vi "testD.vi"(11 "Event Registration Refnum":T1) -> ()   [LabVIEW 2015]
uses:
  D refnum.ctl
panel:
  out "Boolean":bool
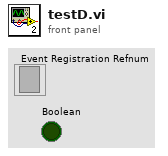
[diagram p1: front panel]
types:
  T1 = typedef "D refnum.ctl" = refnum<event-registration>
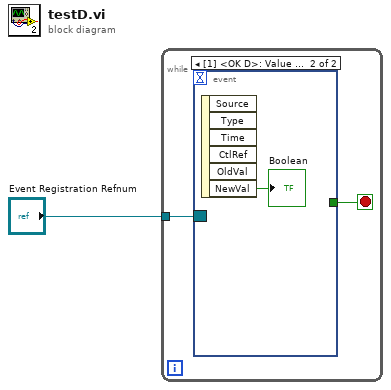
[diagram p0: block diagram]
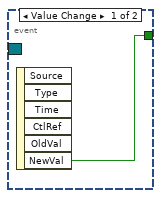
[diagram p2: hidden frame]
diagram:
  n1 = while {
    tunnel: "Event Registration Refnum" -> [w2]
    stop <- w3 stop-if-true
    n2 = event shown="[1] <OK D>: Value Change" {
      selector: w2 -> [_ _]
      dyn-events: _ -> [_ _]
      timeout: _ -> [_ _]
      tunnel: [w4 _] -> w3
      event Value Change {
        n3 = event-data() -> ("NewVal"=w4:bool)  [unwired: 1 in, 5 out]
      }
      event Value Change {
        n4 = event-data() -> ("NewVal"=→"Boolean":bool)  [unwired: 1 in, 5 out]
      }
    }
  }
